vi "氨氮通讯.vi"() -> ()   [LabVIEW 2016, in "斯坦道氨氮.lvlib"]
uses:
  <vilib>/Utility/config.llb/Write Key (String).vi
  <vilib>/Plasmionique/MB Master/MB_Master/MB_Master.lvclass
  <vilib>/Utility/config.llb/NI_LVConfig.lvlib
  <vilib>/Plasmionique/MB Master/MB Master.lvlib
panel:
  out "序列号":string
  out "状态告警区":T1
  out "测量数据区":T2 {"单位" items=["ug/L", "mg/L", "ppm", "mg/m3", "cm", "ppb", "ug/m3", "%", "nmol/mol", "umol/mol", "MPN/L", "MPN/100ml", "ng/m3", "NTU", "无量纲", "ms/cm", "us/cm", "℃", "mV", "万个/L"]}
  out "status":bool
  out "关键参数区":T3
  in  "读关键参数区":bool
  in  "读状态告警区":bool
  in  "读测量数据区":bool
  in  "站号":u16(ring) items=["总磷"=1, "氨氮"=3]
  in  "停止":bool
  in  "启动":bool
  in  "控制命令":u16(ring) items=["启动测量"=1, "标样核查"=2, "零点核查"=3, "跨度核查"=4, "空白测试"=5, "平行样测试"=6, "加标回收"=7, "空白校准"=8, "标样校准"=9, "初始化（清洗）"=10, "停止测试"=11, "仪器重启"=12, "校时"=13, "模式设置"=14, "测量间隔设置"=15]
  in  "控制命令参数":u16[](array[numeric]) format="%04xH"
  in  "VISA Resource":refnum<visa-resource-name>
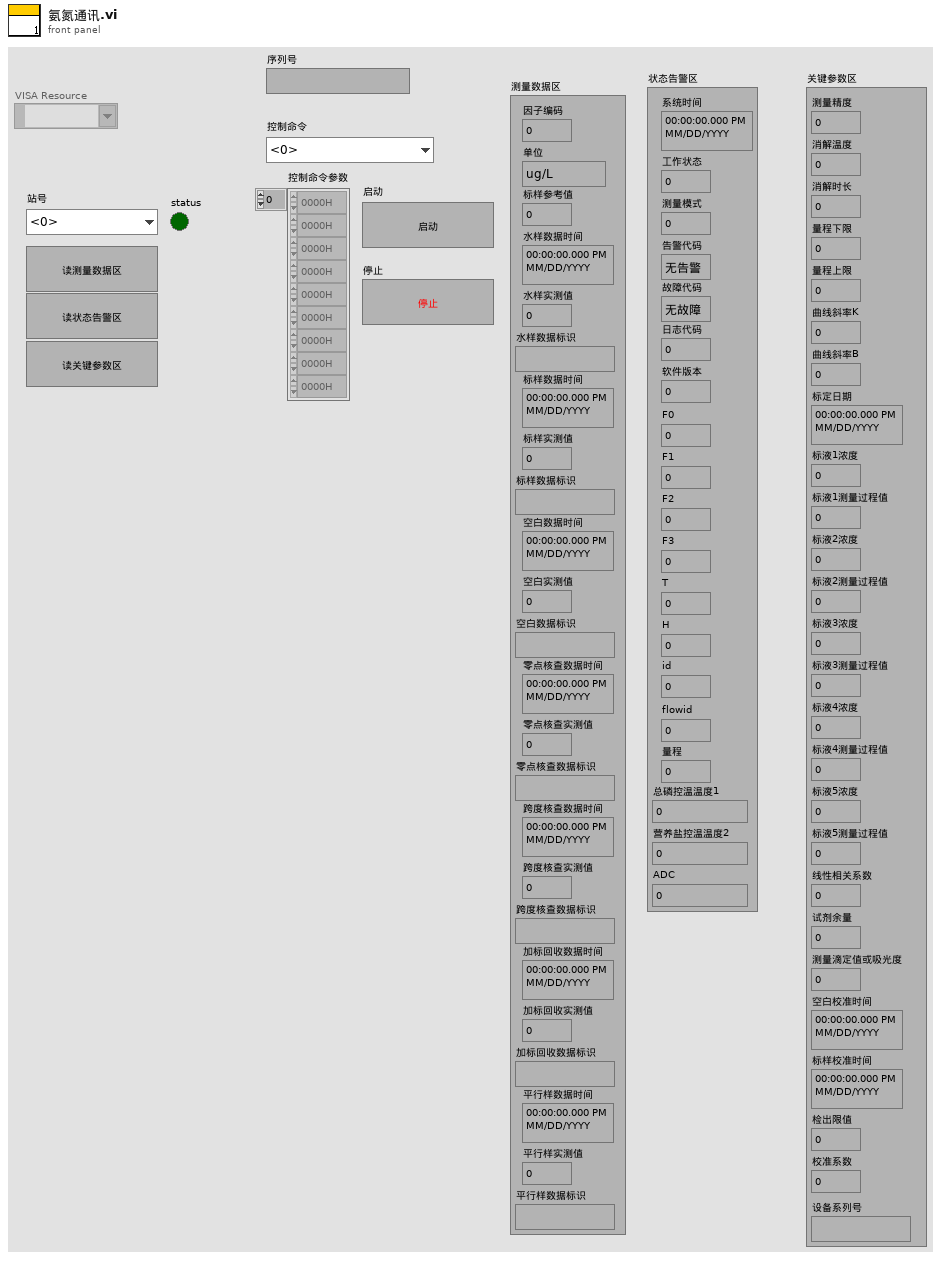
[diagram p1: front panel]
types:
  T1 = cluster{"系统时间":timestamp, "工作状态":u16, "测量模式":u16, "告警代码":enum16{"无告警", "缺试剂告警", "缺水样告警", "缺蒸馏水告警", "缺标液告警", "仪表漏液告警", "标定异常告警", "超量程告警", "加热异常", "低试剂预警", "超上限告警", "超下限告警", "仪表内部其他异常", "滴定异常告警", "电极异常告警", "量程切换告警", "参数设置告警", "PH电极电位异常", "电导率电极异常", "浊度光度异常", "溶解氧电极异常", "溶解氧光强异常", "温度异常告警", "PH异常告警", "溶解氧异常告警", "电导率异常告警", "浊度异常告警", "叶绿素异常告警", "藻密度异常告警", "蓝绿藻异常告警", "ORP异常告警", "氨氮异常告警", "清洁刷异常告警", "SD卡异常告警", "蓝牙异常告警", "Wifi异常告警", "流程异常告警"}, "故障代码":enum16{"无故障", "电机故障", "温度故障", "通讯故障", "滴定故障"}, "日志代码":u16, "软件版本":u16, "F0":sgl, "F1":sgl, "F2":sgl, "F3":sgl, "T":sgl, "H":sgl, "id":u16, "flowid":u16, "量程":u16, "ADC":sgl, "营养盐控温温度2":sgl, "总磷控温温度1":sgl}
  T2 = cluster{"因子编码":u32, "单位":u16, "标样参考值":sgl, "水样数据时间":timestamp, "水样实测值":sgl, "水样数据标识":string, "标样数据时间":timestamp, "标样实测值":sgl, "标样数据标识":string, "空白数据时间":timestamp, "空白实测值":sgl, "空白数据标识":string, "零点核查数据时间":timestamp, "零点核查实测值":sgl, "零点核查数据标识":string, "跨度核查数据时间":timestamp, "跨度核查实测值":sgl, "跨度核查数据标识":string, "加标回收数据时间":timestamp, "加标回收实测值":sgl, "加标回收数据标识":string, "平行样数据时间":timestamp, "平行样实测值":sgl, "平行样数据标识":string}
  T3 = cluster{"测量精度":u16, "消解温度":u16, "消解时长":u16, "量程下限":sgl, "量程上限":sgl, "曲线斜率K":sgl, "曲线斜率B":sgl, "标定日期":timestamp, "标液1浓度":sgl, "标液1测量过程值":sgl, "标液2浓度":sgl, "标液2测量过程值":sgl, "标液3浓度":sgl, "标液3测量过程值":sgl, "标液4浓度":sgl, "标液4测量过程值":sgl, "标液5浓度":sgl, "标液5测量过程值":sgl, "线性相关系数":sgl, "试剂余量":u32, "测量滴定值或吸光度":sgl, "空白校准时间":timestamp, "标样校准时间":timestamp, "检出限值":sgl, "校准系数":sgl, "设备系列号":string}
  T4 = typedef "NI_LVConfig.lvlib/Config Data RefNum.ctl" = refnum<k1>
  T5 = enum8{"Enabled", "Disabled", "Disabled and Grayed Out"}
  T6 = cluster{"系统时间":timestamp, "工作状态":enum16{"空闲", "水样测试", "标样核查", "零点核查", "跨度核查", "空白测试", "平行样测试", "加标回收", "空白校准", "标样校准", "初始化（清洗）"}, "测量模式":enum16{"待机", "连续模式", "周期模式", "定点模式", "受控模式", "手动模式"}, "告警代码":enum16{"无告警", "缺试剂告警", "缺水样告警", "缺蒸馏水告警", "缺标液告警", "仪表漏液告警", "标定异常告警", "超量程告警", "加热异常", "低试剂预警", "超上限告警", "超下限告警", "仪表内部其他异常", "滴定异常告警", "电极异常告警", "量程切换告警", "参数设置告警", "PH电极电位异常", "电导率电极异常", "浊度光度异常", "溶解氧电极异常", "溶解氧光强异常", "温度异常告警", "PH异常告警", "溶解氧异常告警", "电导率异常告警", "浊度异常告警", "叶绿素异常告警", "藻密度异常告警", "蓝绿藻异常告警", "ORP异常告警", "氨氮异常告警", "清洁刷异常告警", "SD卡异常告警", "蓝牙异常告警", "Wifi异常告警", "流程异常告警"}, "故障代码":enum16{"无故障", "电机故障", "温度故障", "通讯故障", "滴定故障"}, "日志代码":u16, "软件版本":u16, "F0":sgl, "F1":sgl, "F2":sgl, "F3":sgl, "T":sgl, "H":sgl, "id":u16, "flowid":u16, "量程":u16, "总磷控温温度1":sgl, "营养盐控温温度2":sgl, "ADC":sgl}
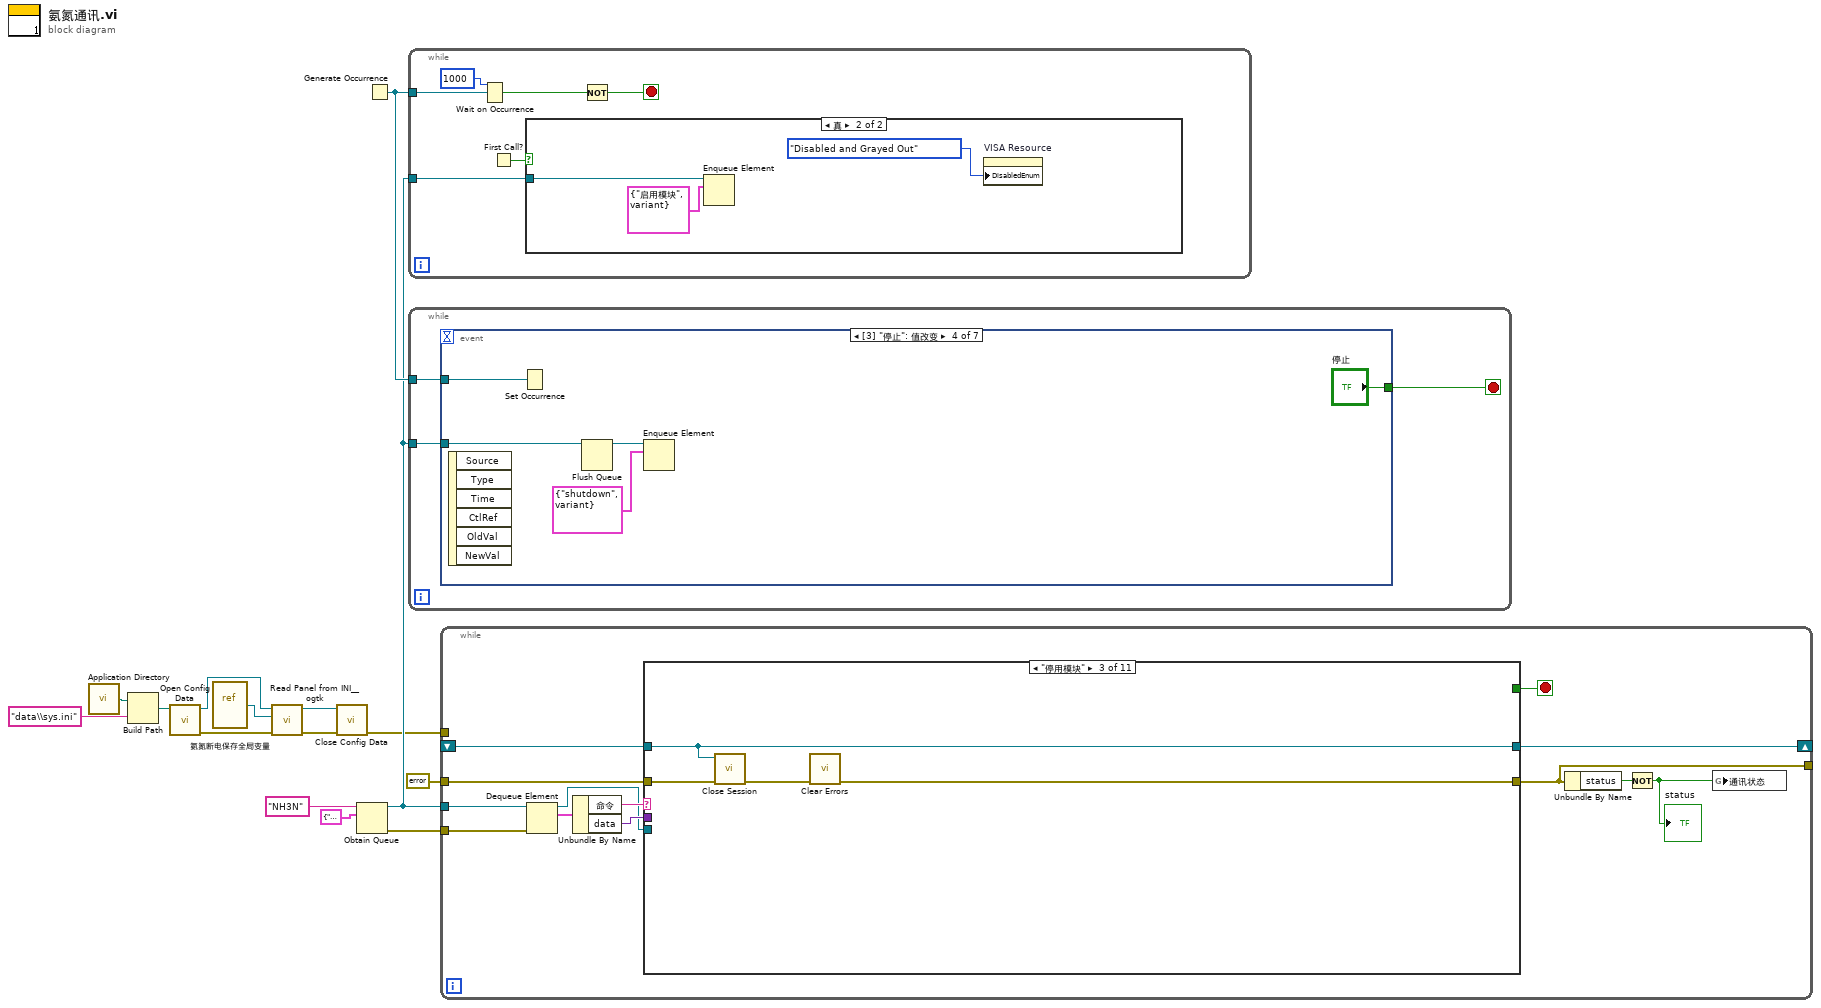
[diagram p0: block diagram]
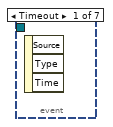
[diagram p3: hidden frame]
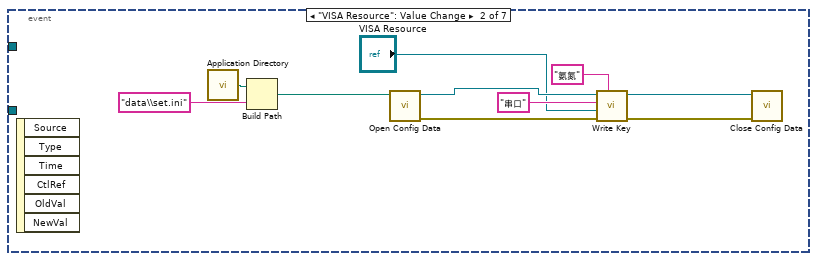
[diagram p4: hidden frame]
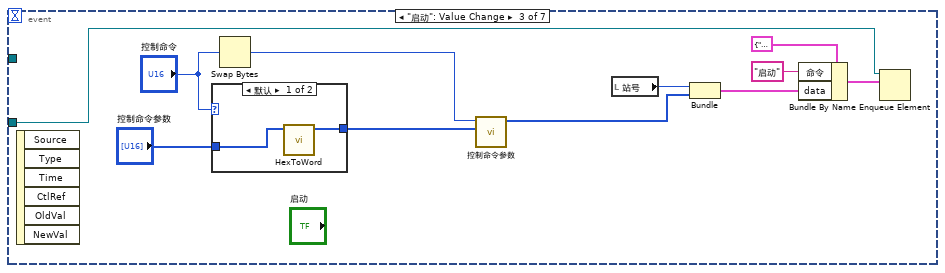
[diagram p5: hidden frame]
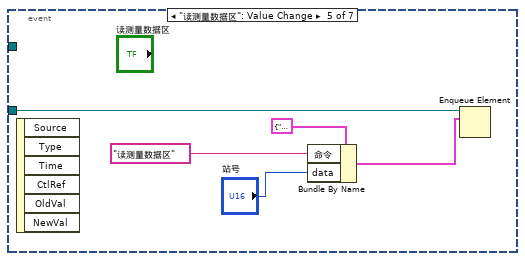
[diagram p7: hidden frame]
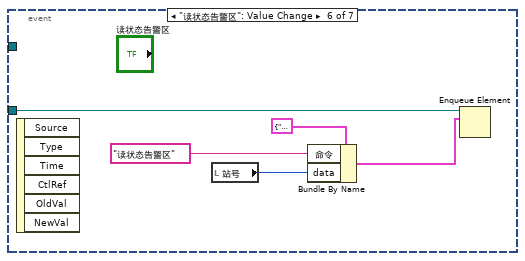
[diagram p8: hidden frame]
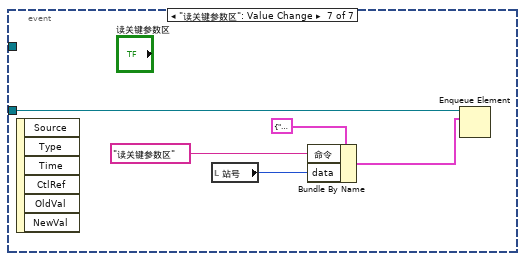
[diagram p9: hidden frame]
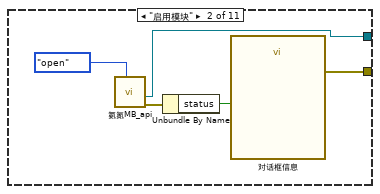
[diagram p11: hidden frame]
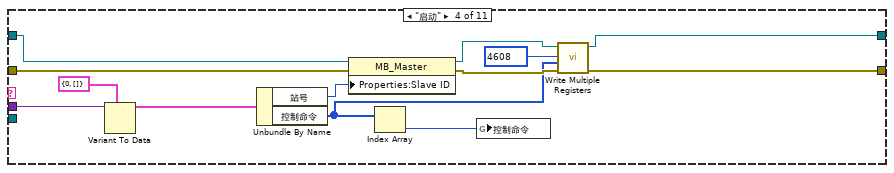
[diagram p12: hidden frame]
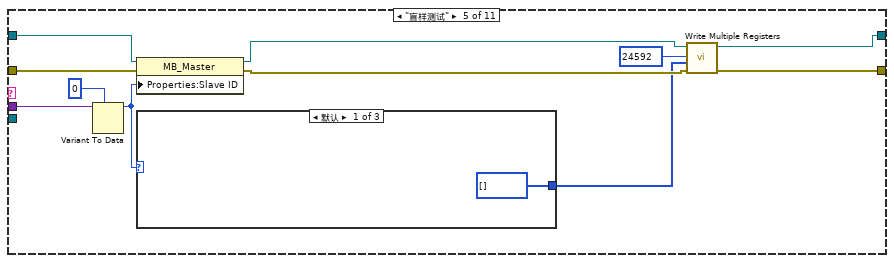
[diagram p13: hidden frame]
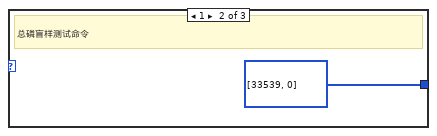
[diagram p14: hidden frame]
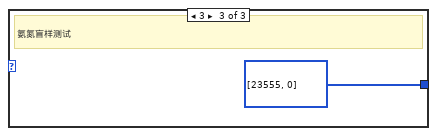
[diagram p15: hidden frame]
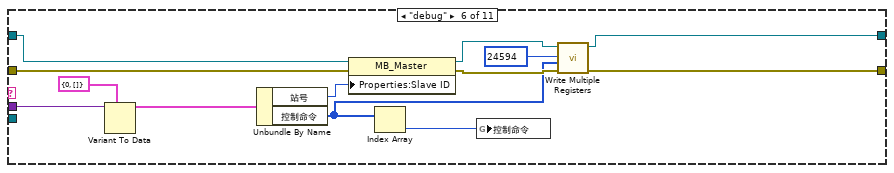
[diagram p16: hidden frame]
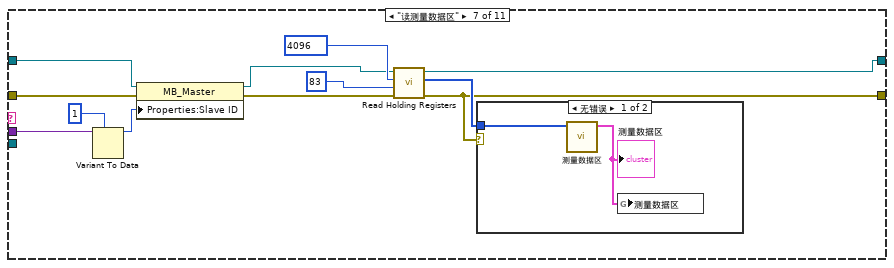
[diagram p17: hidden frame]
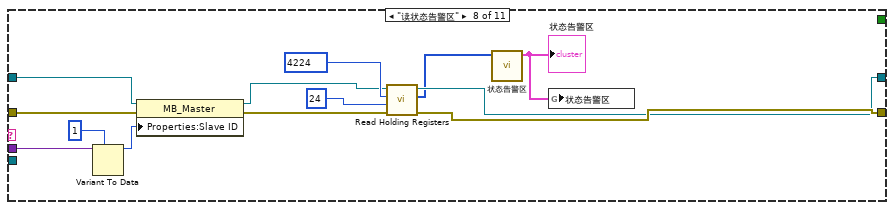
[diagram p19: hidden frame]
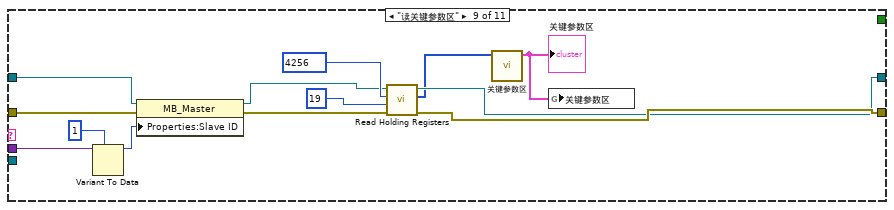
[diagram p20: hidden frame]
diagram:
  n1 = call <vilib>:"Application Directory.vi"() -> ("Application Directory"=w2:path)
  n2 = Build Path(base path=w2, name or relative path="data\\sys.ini" ("名称或相对路径")) -> (appended path=w4:path)
  n3 = call <vilib>:"Open Config Data.vi"("configuration file path"=w4) -> ("error out"=w8:errorcluster, "refnum"=w5:T4)  [unwired: 8 in, 1 out]
  n4 = vi-ref "氨氮断电保存全局变量.vi"() -> (w6:refnum<vi>)
  n5 = call <userlib>:"Read Panel from INI__ogtk.vi"("error in (no error)"=w8, "VI ref"=w6, "refnum"=w5) -> ("error out"=w9:errorcluster, "refnum out"=w7:T4)  [unwired: 7 in]
  n6 = call <vilib>:"Close Config Data.vi"("error in (no error)"=w9, "refnum"=w7) -> ("error out"=w1:errorcluster)  [unwired: 8 in, 1 out]
  n7 = Obtain Queue(name (unnamed)="NH3N" ("名称（未命名）"), element data type=cluster{"命令":string, "data":variant} {"命令"="", "data"=variant}) -> (queue out=w10:refnum<queue>, error out=w13:errorcluster)  [unwired: 3 in, 1 out]
  n8 = Generate Occurrence() -> (w11:refnum<k4>)
  n9 = while {
    tunnel: w11 -> [w21]
    tunnel: w10 -> [w17]
    stop <- w18 stop-if-true
    n10 = Wait on Occurrence(2:w21, 3:1000 ("毫秒超时(-1)")) -> (0:w19:bool)  [unwired: 1 in]
    n11 = First Call?() -> (First Call?: T/F=w16:bool)
    n12 = case shown="真" w16 {
      tunnel: w17 -> [_ w23]
      frame False {
      }
      frame True {
        n13 = Enqueue Element(queue=w23, element=cluster{"命令":string, "data":variant} {"命令"="启用模块", "data"=variant} ("元素")) -> ()  [unwired: 2 in, 3 out]
        n14 = property on="VISA Resource" class="VISAName"("DisabledEnum"=T5."Disabled and Grayed Out" ("禁用")) -> ()  [unwired: 2 in, 2 out]
      }
    }
    n15 = Not(x=w19) -> (.not. x?=w18:bool)
  }
  n16 = while {
    tunnel: w10 -> [w27]
    tunnel: w11 -> [w25]
    stop <- w26 stop-if-true
    n17 = event shown="[3] \"停止\": 值改变" {
      selector: _ -> [_ _ _ _ _ _ _]
      dyn-events: _ -> [_ _ _ _ _ _ _]
      timeout: _ -> [_ _ _ _ _ _ _]
      tunnel: w27 -> [_ _ w48 w55 w61 w66 w71]
      tunnel: [_ _ _ "停止" _ _ _] -> w26
      tunnel: w25 -> [_ _ _ w52 _ _ _]
      event Timeout {
        n18 = event-data() -> ()  [unwired: 1 in, 3 out]
      }
      event "VISA Resource": Value Change {
        n19 = event-data() -> ()  [unwired: 1 in, 6 out]
        n20 = call <vilib>:"Application Directory.vi"() -> ("Application Directory"=w30:path)
        n21 = Build Path(base path=w30, name or relative path="data\\set.ini" ("名称或相对路径")) -> (appended path=w31:path)
        n22 = call <vilib>:"Open Config Data.vi"("configuration file path"=w31) -> ("error out"=w37:errorcluster, "refnum"=w36:T4)  [unwired: 8 in, 1 out]
        n23 = call-poly <vilib>:"Write Key.vi"("section"="氨氮", "error in (no error)"=w37, "value"="VISA Resource", "key"="串口", "refnum"=w36) -> ("error out"=w33:errorcluster, "refnum out"=w29:T4)  [unwired: 4 in, 1 out]
        n24 = call <vilib>:"Close Config Data.vi"("error in (no error)"=w33, "refnum"=w29) -> ()  [unwired: 8 in, 2 out]
      }
      event "启动": Value Change {
        n25 = event-data() -> ()  [unwired: 1 in, 6 out]
        n26 = case shown="默认" "控制命令" {
          tunnel: "控制命令参数" -> [w50 w51]
          tunnel: [w49 w51] -> w38
          frame Default {
            n27 = call "HexToWord.vi"("数组"=w50) -> ("WORD"=w49:u16[])  [unwired: 10 in]
          }
          frame 13 {
          }
        }
        n28 = Swap Bytes(anything="控制命令") -> (byte swapped=w41:u16)
        n29 = call "控制命令参数.vi"("控制命令参数"=w38, "控制命令"=w41) -> ("控制命令输出"=w44:u16[])  [unwired: 9 in]
        n30 = local read "站号"() -> (w43:u16)
        n31 = Bundle("站号"=w43, "控制命令输出"=w44) -> (w42:cluster{"站号":u16, "控制命令输出":u16[]})  [unwired: 1 in]
        n32 = Bundle By Name(cluster=cluster{"命令":string, "data":variant} {"命令"="", "data"=variant} ("元素"), "命令"="启动", "data"=w42) -> (w46:cluster{"命令":string, "data":variant})
        n33 = Enqueue Element(queue=w48, element=w46) -> ()  [unwired: 2 in, 3 out]
      }
      event "停止": Value Change {
        n34 = event-data() -> ()  [unwired: 1 in, 6 out]
        n35 = Set Occurrence(w52) -> ()
        n36 = Flush Queue(queue=w55) -> (queue out=w54:refnum<queue>)  [unwired: 1 in, 2 out]
        n37 = Enqueue Element(queue=w54, element=cluster{"命令":string, "data":variant} {"命令"="shutdown", "data"=variant} ("元素")) -> ()  [unwired: 2 in, 3 out]
      }
      event "读测量数据区": Value Change {
        n38 = event-data() -> ()  [unwired: 1 in, 6 out]
        n39 = Bundle By Name(cluster=cluster{"命令":string, "data":variant} {"命令"="", "data"=variant} ("元素"), "命令"="读测量数据区", "data"="站号") -> (w59:cluster{"命令":string, "data":variant})
        n40 = Enqueue Element(queue=w61, element=w59) -> ()  [unwired: 2 in, 3 out]
      }
      event "读状态告警区": Value Change {
        n41 = event-data() -> ()  [unwired: 1 in, 6 out]
        n42 = local read "站号"() -> (w62:u16)
        n43 = Bundle By Name(cluster=cluster{"命令":string, "data":variant} {"命令"="", "data"=variant} ("元素"), "命令"="读状态告警区", "data"=w62) -> (w64:cluster{"命令":string, "data":variant})
        n44 = Enqueue Element(queue=w66, element=w64) -> ()  [unwired: 2 in, 3 out]
      }
      event "读关键参数区": Value Change {
        n45 = event-data() -> ()  [unwired: 1 in, 6 out]
        n46 = local read "站号"() -> (w67:u16)
        n47 = Bundle By Name(cluster=cluster{"命令":string, "data":variant} {"命令"="", "data"=variant} ("元素"), "命令"="读关键参数区", "data"=w67) -> (w69:cluster{"命令":string, "data":variant})
        n48 = Enqueue Element(queue=w71, element=w69) -> ()  [unwired: 2 in, 3 out]
      }
    }
  }
  n49 = while {
    tunnel: w10 -> [w84]
    tunnel: w13 -> [w83]
    shift-right: [w81] -> _
    shift-left: _ -> [w80]
    tunnel: errorcluster {"status"=FALSE, "code"=0, "source"=""} ("error out") -> [w79]
    tunnel: [w74] -> _
    tunnel: w1 -> [_]
    stop <- w82 stop-if-true
    n50 = Dequeue Element(queue=w84, error in (no error)=w83) -> (queue out=w75:refnum<queue>, element=w77:cluster{"命令":string, "data":variant})  [unwired: 1 in, 2 out]
    n51 = Unbundle By Name(w77) -> ("命令"=w78:string, "data"=w76:variant)
    n52 = case shown="\"停用模块\"" w78 {
      tunnel: w76 -> [_ _ _ w105 w116 w133 w142 w152 w167 w181 _]
      tunnel: w75 -> [_ _ _ _ _ _ _ _ _ _ w194]
      tunnel: [_ _ _ _ _ _ _ _ _ _ TRUE] -> w82
      tunnel: [w85 w88 w92 w108 w119 w135 w147 w161 w174 w188 w190] -> w81
      tunnel: [w86 w90 w93 w107 w118 w134 w136 w162 w175 w189 w191] -> w74
      tunnel: w80 -> [w85 _ w92 w104 w115 w132 w141 w155 w170 w184 w190]
      tunnel: w79 -> [w86 _ w95 w101 w112 w129 w139 w156 w171 w185 w192]
      frame Default {
      }
      frame "启用模块" {
        n53 = call "氨氮MB_api.vi"("STEP"=enum16{"open", "read", "write", "close"}."open") -> ("error out"=w87:errorcluster, "MB session out"=w88:refnum<class "MB_Master.lvclass">)  [unwired: 7 in, 2 out]
        n54 = Unbundle By Name(w87) -> ("status"=w91:bool)
        n55 = call "对话框信息"("Enable"=w91) -> ("error out"=w90:errorcluster)  [unwired: 9 in, 1 out]
      }
      frame "停用模块" {
        n56 = call-dynamic "Close Session.vi"("error in (no error)"=w95, "MB session in"=w92) -> ("error out"=w94:errorcluster)  [unwired: 9 in]
        n57 = call <vilib>:"Clear Errors.vi"("error in (no error)"=w94) -> ("error out"=w93:errorcluster)  [unwired: 5 in, 1 out]
      }
      frame "启动" {
        n58 = Variant To Data(type=cluster{"站号":u16, "控制命令":u16[]} {"站号"=0, "控制命令"=[]} ("输出簇"), Variant=w105) -> (data=w99:cluster{"站号":u16, "控制命令":u16[]})  [unwired: 1 in, 1 out]
        n59 = Unbundle By Name(w99) -> ("站号"=w98:u16, "控制命令"=w96:u16[])
        n60 = property class="MB_Master"(reference=w104, error in=w101, "Properties:Slave ID"=w98) -> (reference out=w103:refnum<class "MB_Master.lvclass">, error out=w102:errorcluster)
        n61 = Index Array(array=w96) -> (element=w97:u16)  [unwired: 1 in]
        n62 = global write "VAR氨氮全局变量.vi" "控制命令"(w97) -> ()
        n63 = call <vilib>:"Write Multiple Registers.vi"("error in (no error)"=w102, "values"=w96, "starting address"=u16 4608, "MB session in"=w103) -> ("error out"=w107:errorcluster, "MB session out"=w108:refnum<class "MB_Master.lvclass">)  [unwired: 6 in]
      }
      frame "盲样测试" {
        n64 = Variant To Data(type=0, Variant=w116) -> (data=w109:i32)  [unwired: 1 in, 1 out]
        n65 = property class="MB_Master"(reference=w115, error in=w112, "Properties:Slave ID"=w109) -> (reference out=w114:refnum<class "MB_Master.lvclass">, error out=w113:errorcluster)
        n66 = case shown="默认" w109 {
          tunnel: [u16[] [] ("values") u16[] [33539, 0] ("values") u16[] [23555, 0] ("values")] -> w111
          frame Default {
          }
          frame 1 {
            # "总磷盲样测试命令"
          }
          frame 3 {
            # "氨氮盲样测试"
          }
        }
        n67 = call <vilib>:"Write Multiple Registers.vi"("error in (no error)"=w113, "values"=w111, "starting address"=u16 24592, "MB session in"=w114) -> ("error out"=w118:errorcluster, "MB session out"=w119:refnum<class "MB_Master.lvclass">)  [unwired: 6 in]
      }
      frame "debug" {
        n68 = Variant To Data(type=cluster{"站号":u16, "控制命令":u16[]} {"站号"=0, "控制命令"=[]} ("输出簇"), Variant=w133) -> (data=w127:cluster{"站号":u16, "控制命令":u16[]})  [unwired: 1 in, 1 out]
        n69 = Unbundle By Name(w127) -> ("站号"=w126:u16, "控制命令"=w124:u16[])
        n70 = property class="MB_Master"(reference=w132, error in=w129, "Properties:Slave ID"=w126) -> (reference out=w131:refnum<class "MB_Master.lvclass">, error out=w130:errorcluster)
        n71 = Index Array(array=w124) -> (element=w125:u16)  [unwired: 1 in]
        n72 = global write "VAR氨氮全局变量.vi" "控制命令"(w125) -> ()
        n73 = call <vilib>:"Write Multiple Registers.vi"("error in (no error)"=w130, "values"=w124, "starting address"=u16 24594, "MB session in"=w131) -> ("error out"=w134:errorcluster, "MB session out"=w135:refnum<class "MB_Master.lvclass">)  [unwired: 6 in]
      }
      frame "读测量数据区" {
        n74 = Variant To Data(type=u8 1 ("Slave ID"), Variant=w142) -> (data=w143:u8)  [unwired: 1 in, 1 out]
        n75 = property class="MB_Master"(reference=w141, error in=w139, "Properties:Slave ID"=w143) -> (reference out=w140:refnum<class "MB_Master.lvclass">, error out=w138:errorcluster)
        n76 = call <vilib>:"Read Holding Registers.vi"("error in (no error)"=w138, "quantity"=u16 83, "starting address"=u16 4096, "MB session in"=w140) -> ("error out"=w136:errorcluster, "Registers"=w137:u16[], "MB session out"=w147:refnum<class "MB_Master.lvclass">)  [unwired: 5 in]
        n77 = case shown="无错误" w136 {
          tunnel: w137 -> [w149 _]
          frame No Error {
            n78 = call "测量数据区.vi"("数组"=w149) -> ("测量数据区"=w148:T2)  [unwired: 10 in]
            "测量数据区" <- w148
            n79 = global write "VAR氨氮全局变量.vi" "测量数据区"(w148) -> ()
          }
          frame Error {
          }
        }
      }
      frame "读状态告警区" {
        n80 = Variant To Data(type=u8 1 ("Slave ID"), Variant=w152) -> (data=w157:u8)  [unwired: 1 in, 1 out]
        n81 = property class="MB_Master"(reference=w155, error in=w156, "Properties:Slave ID"=w157) -> (reference out=w154:refnum<class "MB_Master.lvclass">, error out=w153:errorcluster)
        n82 = call <vilib>:"Read Holding Registers.vi"("error in (no error)"=w153, "quantity"=u16 24, "starting address"=u16 4224, "MB session in"=w154) -> ("error out"=w162:errorcluster, "Registers"=w151:u16[], "MB session out"=w161:refnum<class "MB_Master.lvclass">)  [unwired: 5 in]
        n83 = call "状态告警区.vi"("数组"=w151) -> ("状态告警区"=w150:T6)  [unwired: 10 in]
        "状态告警区" <- w150
        n84 = global write "VAR氨氮全局变量.vi" "状态告警区"(w150) -> ()
      }
      frame "读关键参数区" {
        n85 = Variant To Data(type=u8 1 ("Slave ID"), Variant=w167) -> (data=w165:u8)  [unwired: 1 in, 1 out]
        n86 = property class="MB_Master"(reference=w170, error in=w171, "Properties:Slave ID"=w165) -> (reference out=w169:refnum<class "MB_Master.lvclass">, error out=w168:errorcluster)
        n87 = call <vilib>:"Read Holding Registers.vi"("error in (no error)"=w168, "quantity"=u16 19, "starting address"=u16 4256, "MB session in"=w169) -> ("error out"=w175:errorcluster, "Registers"=w164:u16[], "MB session out"=w174:refnum<class "MB_Master.lvclass">)  [unwired: 5 in]
        n88 = call "关键参数区.vi"("数组"=w164) -> ("关键参数区"=w163:T3)  [unwired: 10 in]
        "关键参数区" <- w163
        n89 = global write "VAR氨氮全局变量.vi" "关键参数区"(w163) -> ()
      }
      frame "读序列号" {
        n90 = Variant To Data(type=u8 1 ("Slave ID"), Variant=w181) -> (data=w179:u8)  [unwired: 1 in, 1 out]
        n91 = property class="MB_Master"(reference=w184, error in=w185, "Properties:Slave ID"=w179) -> (reference out=w183:refnum<class "MB_Master.lvclass">, error out=w182:errorcluster)
        n92 = call <vilib>:"Read Holding Registers.vi"("error in (no error)"=w182, "quantity"=u16 6, "starting address"=u16 3, "MB session in"=w183) -> ("error out"=w189:errorcluster, "Registers"=w178:u16[], "MB session out"=w188:refnum<class "MB_Master.lvclass">)  [unwired: 5 in]
        n93 = call "HexToString.vi"("数组"=w178) -> ("STRING"=w177:string[])  [unwired: 10 in]
        n94 = Index Array(array=w177) -> (element=w176:string)  [unwired: 1 in]
        "序列号" <- w176
        n95 = global write "VAR氨氮全局变量.vi" "序列号"(w176) -> ()
      }
      frame "shutdown" {
        n96 = call-dynamic "Close Session.vi"("error in (no error)"=w192, "MB session in"=w190) -> ("error out"=w191:errorcluster)  [unwired: 9 in]
        n97 = Flush Queue(queue=w194) -> (queue out=w193:refnum<queue>)  [unwired: 1 in, 2 out]
        n98 = Release Queue(queue=w193) -> ()  [unwired: 2 in, 3 out]
      }
    }
    n99 = Unbundle By Name(w74) -> ("status"=w73:bool)
    n100 = Not(x=w73) -> (.not. x?=w72:bool)
    "status" <- w72
    n101 = global write "VAR氨氮全局变量.vi" "通讯状态"(w72) -> ()
  }
